vi "Read LastByte.vi"(8 "error in":errorcluster, 11 "Buffer":refnum<data-value>) -> (0 "error out":errorcluster, 1 "found":bool, 2 "byte":u8 format="%02x", 3 "Buffer":refnum<data-value>)   [LabVIEW 2013, in "ByteBuffer.lvclass"]
doc: "This VI returns data from the ring buffer starting from the oldest data and ending with the newest.\n\nThe data is duplicated at the output so this VI allocates new place in the memory for the output."
uses:
  ByteBuffer.lvclass
  VariantBuffer/VariantBuffer.lvclass
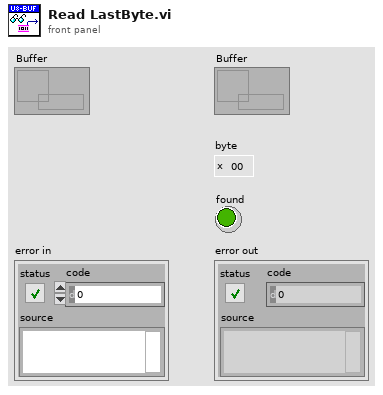
[diagram p1: front panel]
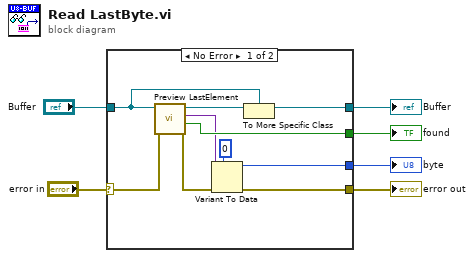
[diagram p0: block diagram]
diagram:
  n1 = case shown="No Error" "error in" {
    selector: "error in" -> [w15 w17]
    tunnel: "Buffer" -> [w7 w18]
    tunnel: [w8 w18] -> w5
    tunnel: [w9 w17] -> w3
    tunnel: [w12 _] -> w1
    tunnel: [w14 _] -> w2
    frame No Error {
      n2 = call "Preview LastElement.vi"("error in"=w15, "Buffer in"=w7) -> ("error out"=w10:errorcluster, "found"=w14:bool, "element"=w13:variant, "Buffer"=w16:refnum<data-value>)  [unwired: 6 in]
      n3 = Variant To Data(error in=w10, type=u8 0 ("byte"), Variant=w13) -> (data=w12:u8, error out=w9:errorcluster)
      n4 = To More Specific Class(target class=w7, reference=w16) -> (specific class reference=w8:refnum<data-value>)  [unwired: 1 in, 1 out]
    }
    frame Error {
    }
  }
  "error out" <- w3
  "Buffer" <- w5
  "byte" <- w1
  "found" <- w2
